vi "SSH-Hostname-Command.vi"(5 "DUT Number In (start at 0)":i32, 7 "New IP (to assign)":string="44.44.55.20", 9 "Select DUT Type (input)":T1, 11 "error in":errorcluster, 12 "Generator-Original IP":string="44.44.55.100", 14 "Remote-Original IP":string="44.44.55.101") -> (3 "IP Config Errors":string, 6 "DUT NumberOut":i32, 10 "New IP (Out)":string="44.44.51.20", 15 "error out":errorcluster)   [LabVIEW 2012]
uses:
  C:/_SJM/test_apps/dev/90131441_Ampere_Run_In/Controls/DUT-Type-Select.ctl
  <vilib>/Utility/error.llb/whitespace.ctl
panel:
  out "appended script file":path
  out "Command Executed":string
  in  "Protocol":u16(ring)=2 items=["Telnet", "Rlogin", "SSH", "RAW"]
  out "Command Return Value(s)":string
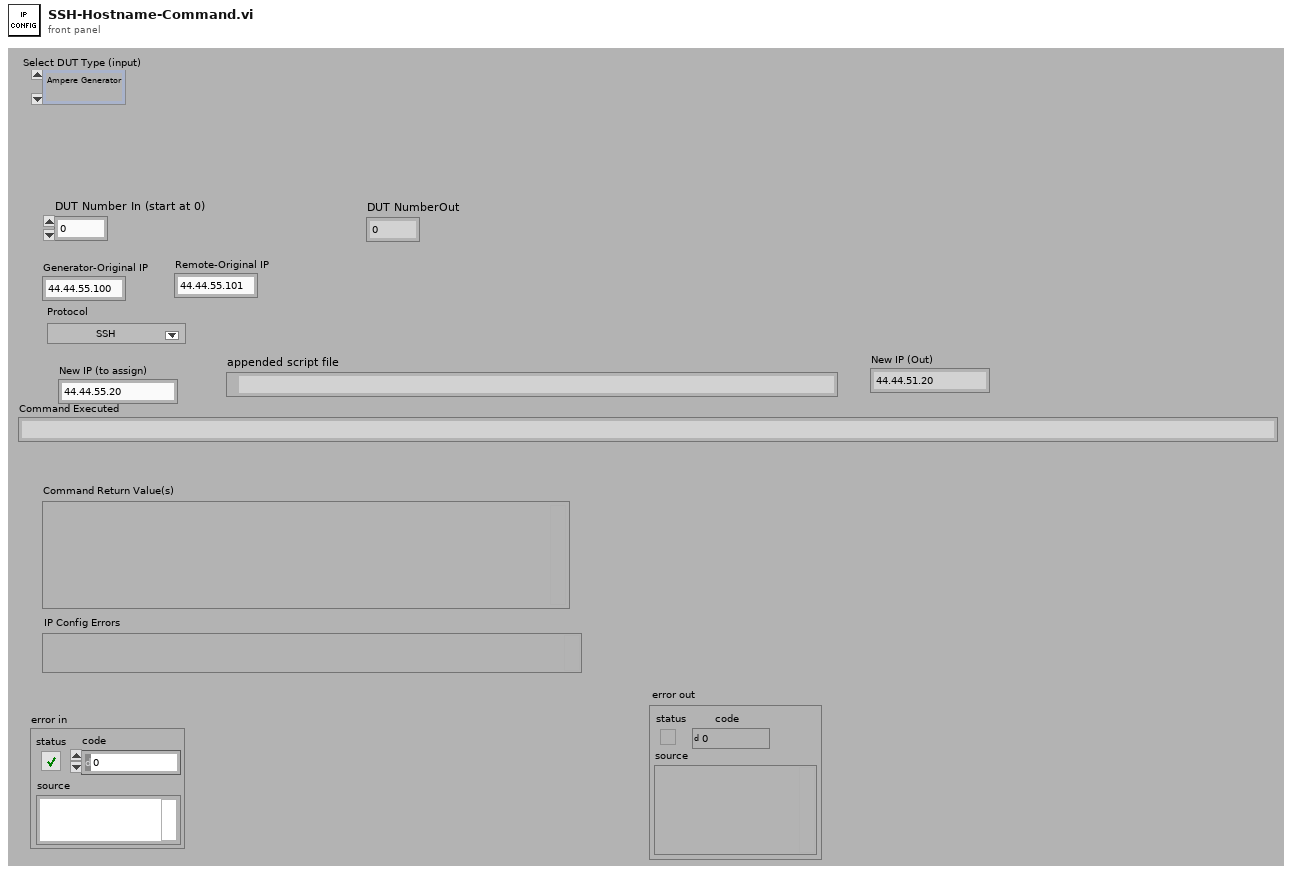
[diagram p1: front panel]
types:
  T1 = typedef "DUT-Type-Select.ctl" = enum16{"Ampere Generator", "Ampere Remote"}
  T2 = enum16{"open", "replace", "create", "open or create", "replace or create", "replace or create with confirmation"}
  T3 = typedef "whitespace.ctl" = u16
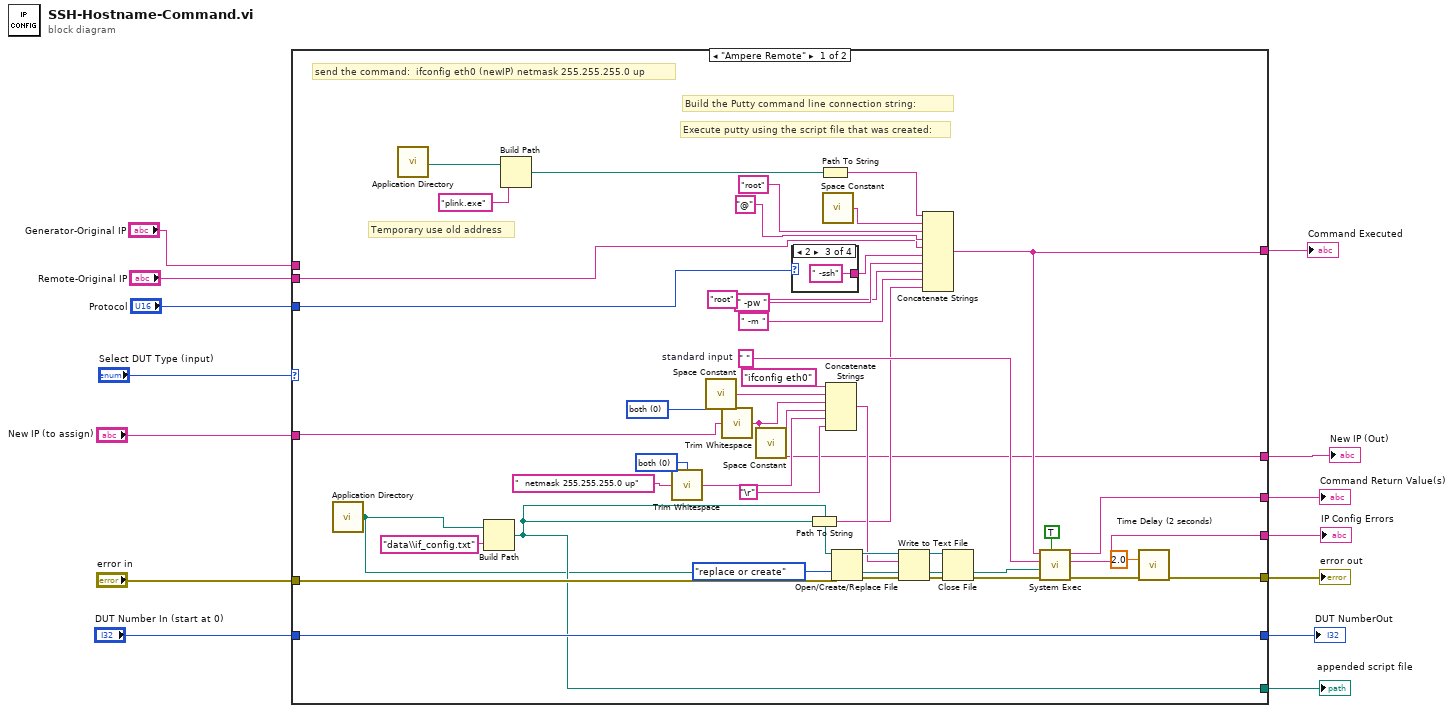
[diagram p0: block diagram]
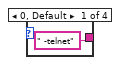
[diagram p2: hidden frame]
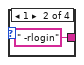
[diagram p3: hidden frame]
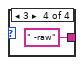
[diagram p4: hidden frame]
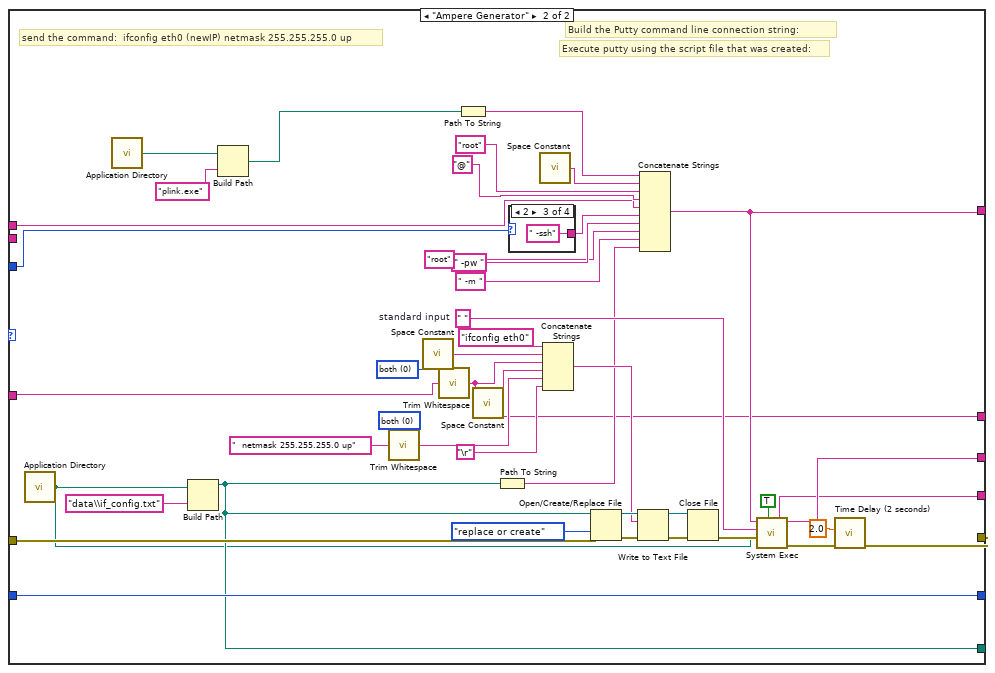
[diagram p5: hidden frame]
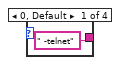
[diagram p6: hidden frame]
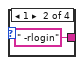
[diagram p7: hidden frame]
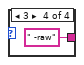
[diagram p8: hidden frame]
diagram:
  n1 = case shown="\"Ampere Remote\"" "Select DUT Type (input)" {
    tunnel: [w58 w106] -> w14
    tunnel: "Generator-Original IP" -> [_ w96]
    tunnel: [w24 w73] -> w13
    tunnel: [w44 w91] -> w12
    tunnel: "error in" -> [w42 w90]
    tunnel: [w31 w79] -> w10
    tunnel: [w25 w74] -> w9
    tunnel: "DUT Number In (start at 0)" -> [w25 w74]
    tunnel: [w16 w63] -> w6
    tunnel: "New IP (to assign)" -> [w22 w72]
    tunnel: [w21 w68] -> w4
    tunnel: "Protocol" -> [w20 w71]
    tunnel: "Remote-Original IP" -> [w15 _]
    frame "Ampere Remote" {
      w33 = T3 0 items=["both", "start of string", "end of string"] ("location (both)")
      w37 = T3 0 items=["both", "start of string", "end of string"] ("location (both)")
      w51 = " "  # standard input
      # "Temporary use old address"
      # "send the command:  ifconfig eth0 (newIP) netmask 255.255.255.0 up"
      # "Execute putty using the script file that was created:"
      # "Build the Putty command line connection string:"
      n2 = call <vilib>:"Application Directory.vi"() -> ("Application Directory"=w17:path)
      n3 = call <vilib>:"Application Directory.vi"() -> ("Application Directory"=w19:path)
      n4 = Build Path(base path=w17, name or relative path="data\\if_config.txt") -> (appended path=w21:path)
      n5 = Build Path(base path=w19, name or relative path="plink.exe") -> (appended path=w29:path)
      n6 = call <vilib>:"Trim Whitespace.vi"("string"="  netmask 255.255.255.0 up", "location (both)"=w33) -> ("trimmed string"=w34:string)
      n7 = call <vilib>:"Space Constant.vi"() -> ("String"=w39:string)
      n8 = call <vilib>:"Trim Whitespace.vi"("string"=w22, "location (both)"=w37) -> ("trimmed string"=w16:string)
      n9 = call <vilib>:"Space Constant.vi"() -> ("String"=w38:string)
      n10 = case shown="2" w20 {
        tunnel: [" -telnet" " -rlogin" " -ssh" " -raw"] -> w48
        frame 0, Default {
        }
        frame 1 {
        }
        frame 2 {
        }
        frame 3 {
        }
      }
      n11 = Path To String(path=w21) -> (string=w26:string)
      n12 = Path To String(path=w29) -> (string=w18:string)
      n13 = call <vilib>:"Space Constant.vi"() -> ("String"=w28:string)
      n14 = Concatenate Strings("ifconfig eth0" ("string"), w39, w16, w38, w34, "\r") -> (w40:string)
      n15 = Open/Create/Replace File(file path (use dialog)=w21, error in=w42, operation (0:open)=T2."replace or create") -> (refnum out=w54:refnum<file>, error out=w53:errorcluster)  [unwired: 3 in, 1 out]
      n16 = Write to Text File(file (use dialog)=w54, text=w40, error in=w53) -> (refnum out=w57:refnum<file>, error out=w56:errorcluster)  [unwired: 2 out]
      n17 = Concatenate Strings(w18, w28, "root" ("Username"), "@" ("string"), w15, w48, " -pw " ("string"), "root" ("Password"), " -m " ("string"), w26) -> (w24:string)
      n18 = Close File(refnum=w57, error in=w56) -> (error out=w55:errorcluster)  [unwired: 1 out]
      n19 = call <vilib>:"System Exec.vi"("run minimized? (F)"=TRUE ("Hide DOS\nWindow?"), "error in (no error)"=w55, "working directory"=w17, "standard input"=w51, "command line"=w24) -> ("error out"=w32:errorcluster, "standard error"=w44:string, "standard output"=w58:string)  [unwired: 1 in, 3 out]
      n20 = call "Time Delay (2 seconds)"("error in (no error)"=w32, "Delay Time (s)"=2.0) -> ("error out"=w31:errorcluster)  [unwired: 9 in]
    }
    frame "Ampere Generator" {
      w81 = T3 0 items=["both", "start of string", "end of string"] ("location (both)")
      w85 = T3 0 items=["both", "start of string", "end of string"] ("location (both)")
      w99 = " "  # standard input
      # "send the command:  ifconfig eth0 (newIP) netmask 255.255.255.0 up"
      # "Execute putty using the script file that was created:"
      # "Build the Putty command line connection string:"
      n21 = call <vilib>:"Application Directory.vi"() -> ("Application Directory"=w64:path)
      n22 = call <vilib>:"Application Directory.vi"() -> ("Application Directory"=w70:path)
      n23 = Build Path(base path=w64, name or relative path="data\\if_config.txt") -> (appended path=w68:path)
      n24 = Build Path(base path=w70, name or relative path="plink.exe") -> (appended path=w69:path)
      n25 = call <vilib>:"Trim Whitespace.vi"("string"="  netmask 255.255.255.0 up", "location (both)"=w81) -> ("trimmed string"=w82:string)
      n26 = call <vilib>:"Space Constant.vi"() -> ("String"=w87:string)
      n27 = call <vilib>:"Trim Whitespace.vi"("string"=w72, "location (both)"=w85) -> ("trimmed string"=w63:string)
      n28 = Path To String(path=w69) -> (string=w67:string)
      n29 = call <vilib>:"Space Constant.vi"() -> ("String"=w86:string)
      n30 = Path To String(path=w68) -> (string=w66:string)
      n31 = case shown="2" w71 {
        tunnel: [" -telnet" " -rlogin" " -ssh" " -raw"] -> w95
        frame 0, Default {
        }
        frame 1 {
        }
        frame 2 {
        }
        frame 3 {
        }
      }
      n32 = call <vilib>:"Space Constant.vi"() -> ("String"=w76:string)
      n33 = Concatenate Strings("ifconfig eth0" ("string"), w87, w63, w86, w82, "\r") -> (w88:string)
      n34 = Open/Create/Replace File(file path (use dialog)=w68, error in=w90, operation (0:open)=T2."replace or create") -> (refnum out=w102:refnum<file>, error out=w101:errorcluster)  [unwired: 3 in, 1 out]
      n35 = Write to Text File(file (use dialog)=w102, text=w88, error in=w101) -> (refnum out=w105:refnum<file>, error out=w104:errorcluster)  [unwired: 2 out]
      n36 = Concatenate Strings(w67, w76, "root" ("Username"), "@" ("string"), w96, w95, " -pw " ("string"), "root" ("Password"), " -m " ("string"), w66) -> (w73:string)
      n37 = Close File(refnum=w105, error in=w104) -> (error out=w103:errorcluster)  [unwired: 1 out]
      n38 = call <vilib>:"System Exec.vi"("run minimized? (F)"=TRUE ("Hide DOS\nWindow?"), "error in (no error)"=w103, "working directory"=w64, "standard input"=w99, "command line"=w73) -> ("error out"=w80:errorcluster, "standard error"=w91:string, "standard output"=w106:string)  [unwired: 1 in, 3 out]
      n39 = call "Time Delay (2 seconds)"("error in (no error)"=w80, "Delay Time (s)"=2.0) -> ("error out"=w79:errorcluster)  [unwired: 9 in]
    }
  }
  "Command Return Value(s)" <- w14
  "IP Config Errors" <- w12
  "Command Executed" <- w13
  "error out" <- w10
  "DUT NumberOut" <- w9
  "New IP (Out)" <- w6
  "appended script file" <- w4
